vi "DSF.Execution.Builder.Run.vi"(8 "error in (no error)":errorcluster, 11 "Builder in":refnum<class "DSF.Execution.Builder.lvclass">) -> (0 "error out":errorcluster, 3 "Builder out":refnum<class "DSF.Execution.Builder.lvclass">)   [LabVIEW 2016, in "DSF.Engine.lvlib" / "DSF.Execution.Builder.lvclass"]
uses:
  DSF.Execution.Builder.lvclass
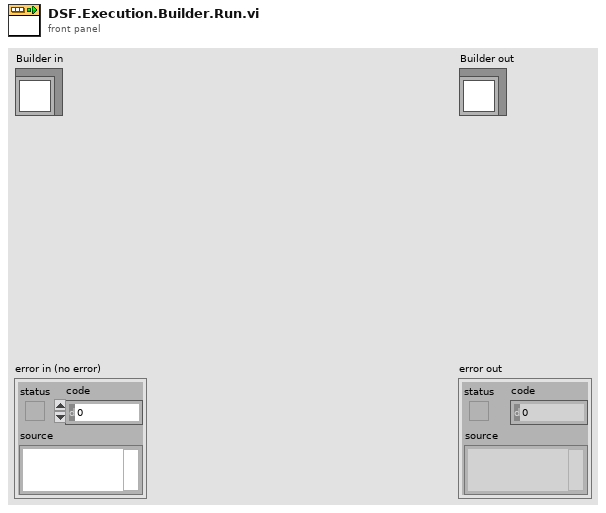
[diagram p1: front panel]
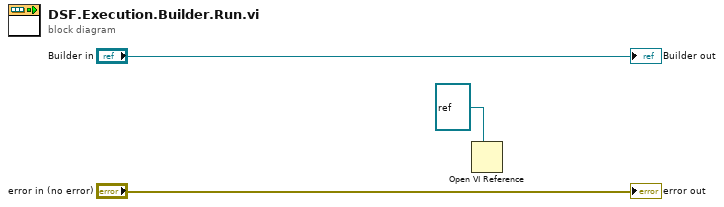
[diagram p0: block diagram]
diagram:
  n1 = Open VI Reference(type specifier VI Refnum (for type only)=refnum<vi> refnum) -> ()  [unwired: 5 in, 2 out]
  "error out" <- "error in (no error)"
  "Builder out" <- "Builder in"
